vi "mod_IQ Impairments Axis Shear.vi"(0 "Input Complex Waveform":T1 {"Y" format="%.3f"; "dt" format="%^.2e"; "t0" format="%.4f"}, 2 "IQ Gain Imbalance, dB":dbl format="%.2f", 3 "Quadrature Skew, degrees":dbl format="%.2f", 11 "error in (no error)":errorcluster) -> (4 "Output Complex Waveform":T1 {"Y" format="%.3f"; "dt" format="%^.2e"; "t0" format="%.4f"}, 15 "error out":errorcluster)   [LabVIEW 2020, in "niDMT.lvlib"]
doc: "Performs the Gain Imbalance operation for IQ Impairment of an Input Data Waveform."
uses:
  <vilib>/addons/Modulation/niDMT.lvlib
  <vilib>/addons/Modulation/Analog/controls/Complex Data Waveform.ctl
  <vilib>/addons/Modulation/niAMT.lvlib
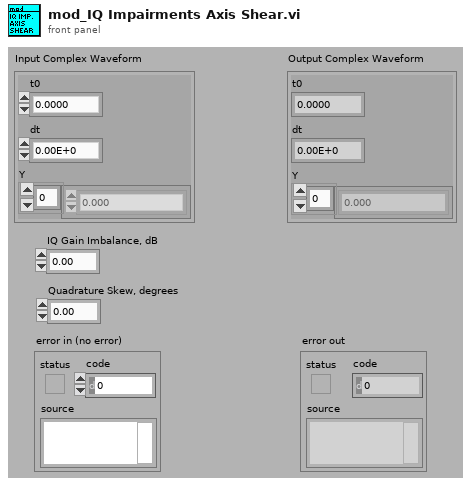
[diagram p1: front panel]
types:
  T1 = typedef "niAMT.lvlib/Complex Data Waveform.ctl" = cluster{"t0":dbl, "dt":dbl, "Y":cdb[]}
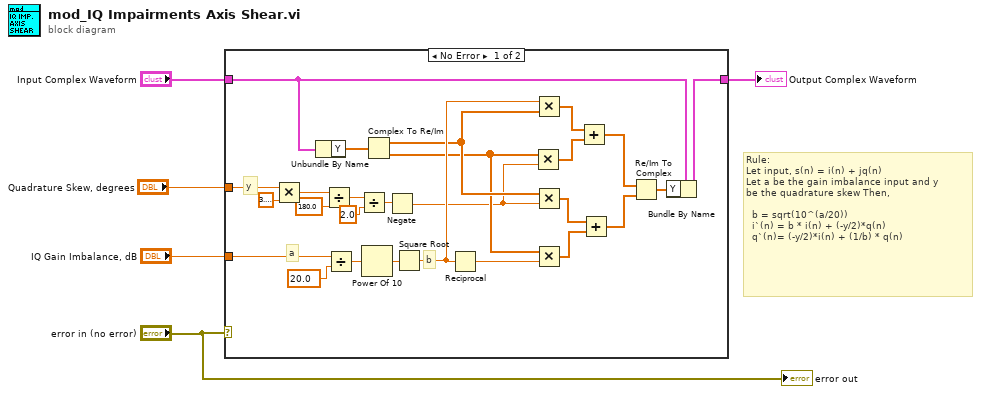
[diagram p0: block diagram]
diagram:
  # "Rule:\nLet input, s(n) = i(n) + jq(n)\nLet a be the gain imbalance input and y \nbe the quadrature skew Then,\n\n  b = sqrt(10^(a/20))\n  i`(n) = b * i(n) + (-y/2)*q(n)\n  q`(n)= (-y/2)*i(n) + (1/b) * q(n)"
  n1 = case shown="No Error" "error in (no error)" {
    tunnel: "IQ Gain Imbalance, dB" -> [w27 _]
    tunnel: "Input Complex Waveform" -> [w29 w32]
    tunnel: [w28 w32] -> w2
    tunnel: "Quadrature Skew, degrees" -> [w20 _]
    frame No Error {
      # "y"
      # "a"
      # "b"
      n2 = Multiply(x=w20, y=3.141592653589793) -> (x*y=w19:dbl)
      n3 = Unbundle By Name(w29) -> ("Y"=w26:cdb[])
      n4 = Divide(x=w19, y=180.0) -> (x/y=w16:dbl)
      n5 = Divide(x=w27, y=20.0) -> (x/y=w30:dbl)
      n6 = Divide(x=w16, y=2.0) -> (x/y=w14:dbl)
      n7 = Power Of 10(x=w30) -> (10^x=w13:dbl)
      n8 = Complex To Re/Im(x + iy=w26) -> (x=w11:dbl[], y=w7:dbl[])
      n9 = Negate(x=w14) -> (-x=w6:dbl)
      n10 = Square Root(x=w13) -> (sqrt(x)=w12:dbl)
      n11 = Reciprocal(x=w12) -> (1/x=w10:dbl)
      n12 = Multiply(x=w7, y=w6) -> (x*y=w9:dbl[])
      n13 = Multiply(x=w12, y=w11) -> (x*y=w23:dbl[])
      n14 = Multiply(x=w11, y=w6) -> (x*y=w8:dbl[])
      n15 = Multiply(x=w7, y=w10) -> (x*y=w24:dbl[])
      n16 = Add(x=w23, y=w9) -> (x+y=w22:dbl[])
      n17 = Add(x=w8, y=w24) -> (x+y=w21:dbl[])
      n18 = Re/Im To Complex(1:w21, 2:w22) -> (0:w25:cdb[])
      n19 = Bundle By Name(cluster=w29, "Y"=w25) -> (w28:T1)
    }
    frame Error {
    }
  }
  "Output Complex Waveform" <- w2
  "error out" <- "error in (no error)"
